vi "LHF.DB.Mongo.Collection.Find.vi"(8 "error in (no error)":errorcluster, 9 "query":refnum<k24>, 10 "Collection":string, 11 "LHF.DB.Mongo in":refnum<class "LHF.DB.Mongo.lvclass">) -> (0 "error out":errorcluster, 2 "Documents":string[](array[string]), 3 "LHF.DB.Mongo out":refnum<class "LHF.DB.Mongo.lvclass">, 5 "ObjectIDs":string[](array[string]))   [LabVIEW 2013, in "LHF.DB.Mongo.lvclass"]
uses:
  LHF.DB.Mongo.lvclass
  C:/Users/schim/Desktop/Projetos/LabVIEW-MongoDB/src/Driver/MongoDB.Driver.dll
  Driver/MongoDB.Driver.dll
panel:
  in  "Extract _id":bool=TRUE
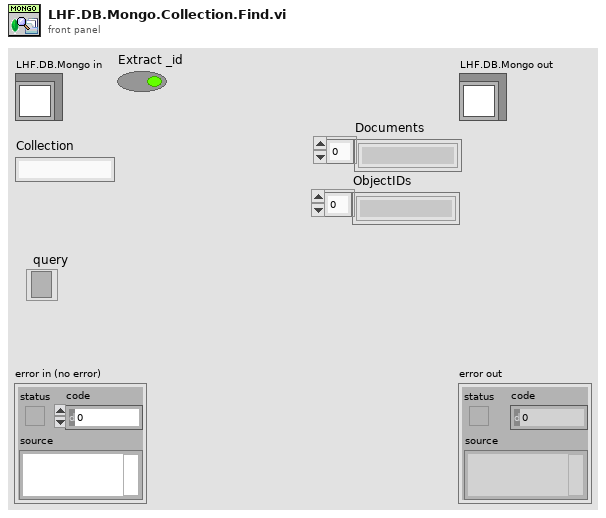
[diagram p1: front panel]
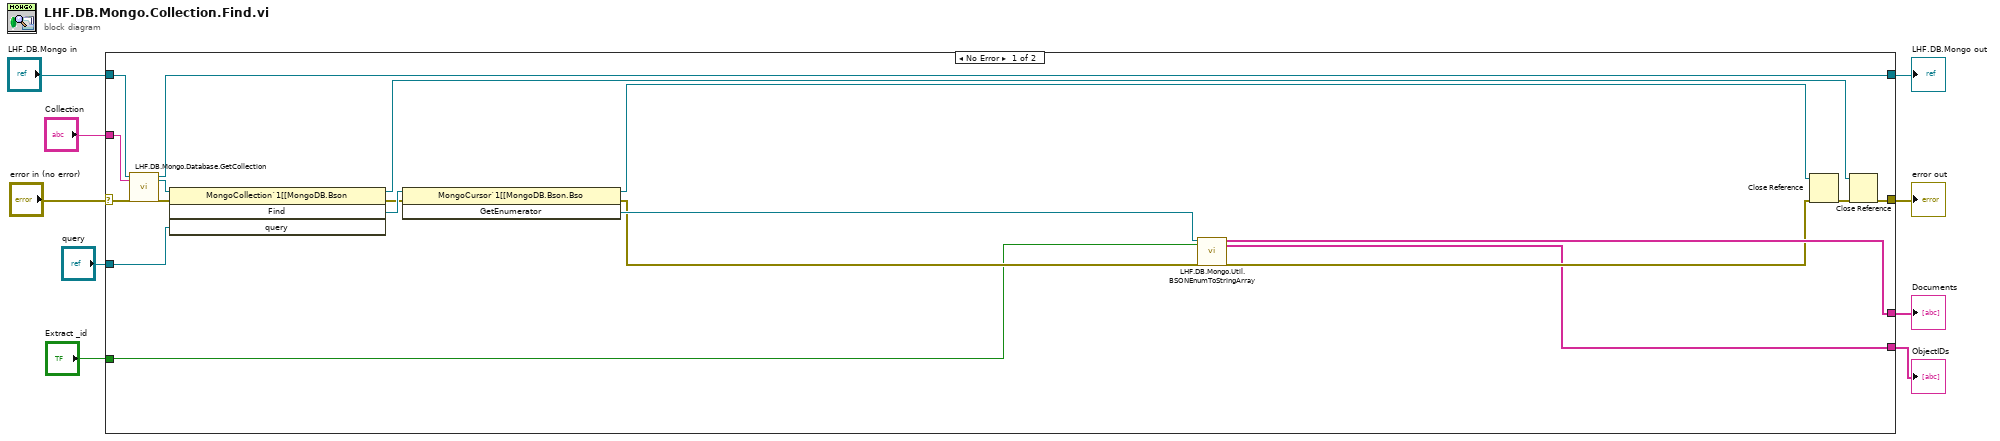
[diagram p0: block diagram]
diagram:
  n1 = case shown="No Error" "error in (no error)" {
    selector: "error in (no error)" -> [w14 w30]
    tunnel: [w17 w30] -> w8
    tunnel: [w27 w29] -> w6
    tunnel: "LHF.DB.Mongo in" -> [w26 w29]
    tunnel: "Collection" -> [w28 _]
    tunnel: [w23 _] -> w4
    tunnel: "query" -> [w13 _]
    tunnel: [w11 _] -> w2
    tunnel: "Extract _id" -> [w10 _]
    frame No Error {
      n2 = call "LHF.DB.Mongo.Database.GetCollection.vi"("LHF.DB.Mongo in"=w26, "collectionName"=w28, "error in (no error)"=w14) -> ("LHF.DB.Mongo in"=w27:refnum<class "LHF.DB.Mongo.lvclass">, "MongoCollection"=w15:refnum<k24>, "error out"=w12:errorcluster)  [unwired: 14 in]
      n3 = invoke class="MongoCollection`1[[MongoDB.Bson" method="Find"(reference=w15, error in=w12, "query"=w13) -> (reference out=w19:refnum<k24>, error out=w21:errorcluster, "Find"=w25:refnum<k24>)  [unwired: 1 in, 1 out]
      n4 = invoke class="MongoCursor`1[[MongoDB.Bson.Bso" method="GetEnumerator"(reference=w25, error in=w21) -> (reference out=w20:refnum<k24>, error out=w22:errorcluster, "GetEnumerator"=w24:refnum<k24>)  [unwired: 1 in]
      n5 = call "LHF.DB.Mongo.Util.BSONEnumToStringArray.vi"("BsonENUM"=w24, "Extract ObjectID"=w10, "error in (no error)"=w22) -> ("Documents"=w23:string[], "ObjectIDs"=w11:string[], "error out"=w16:errorcluster)  [unwired: 14 in]
      n6 = Close Reference(reference=w20, error in (no error)=w16) -> (error out=w18:errorcluster)
      n7 = Close Reference(reference=w19, error in (no error)=w18) -> (error out=w17:errorcluster)
    }
    frame Error {
    }
  }
  "error out" <- w8
  "LHF.DB.Mongo out" <- w6
  "Documents" <- w4
  "ObjectIDs" <- w2
